vi "choosePlayVSS.vi"(8 "error in (no error)":errorcluster, 11 "Game in":refnum<class "Game.lvclass">) -> (0 "error out":errorcluster, 3 "Game out":refnum<class "Game.lvclass">)   [LabVIEW 2018, in "Game.lvclass"]
uses:
  Game.lvclass
  Referee_class/command_interpreted.ctl
  Game.lvclass/Game.ctl
  Referee_class/Referee.lvclass/Referee.ctl
  HaltPlay_class/HaltPlay.lvclass
  PreparePenaltyAllyPlayVSS_class/PreparePenaltyAllyPlayVSS.lvclass
  Read KeeperTeam.vi
  Read Referee.vi
  Referee_class/Read command_interpreted.vi
  Read AllyRef.vi
  Write AllyRef.vi
  Write KeeperTeam.vi
  Ally_class/Ally.lvclass
  C:/Users/anton/Desktop/RoboIme/vsspssl/SSL_AI/Team_class/Team.lvclass
  Referee_class/Referee.lvclass
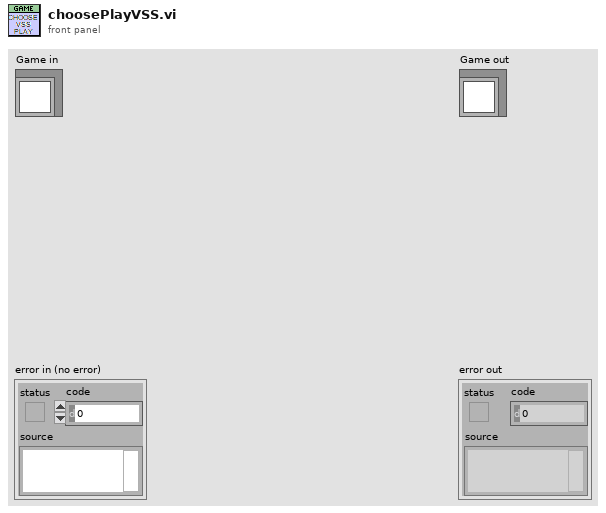
[diagram p1: front panel]
types:
  T1 = typedef "command_interpreted.ctl" = enum16{"Goal Ally", "Goal Enemy", "Ball Placement Enemy", "Ball Placement Ally", "Normal Half Time", "Extra Time  Break", "Extra Half Time", "None", "Post Game", "PKA Normal Start", "Prepare Kickoff Ally", "PKE Normal Start", "Prepare Kickoff Enemy", "Force Start", "Halt", "Timeout", "Prepare Penalty Ally", "Prepare Penalty Enemy", "PPA NormalStart", "PPE Normal Start", "Indirect Free Ally", "Direct Free Enemy", "Direct Free Ally", "Indirect Free Enemy", "Stop"}
  T2 = enum16{"Timeout", "NormalGame", "KickPenaltyAlly", "PenaltyEnemy", "BallChallenge", "PreparePenaltyAlly", "Halt"}
  T3 = enum16{"Timeout", "NormalGame", "KickPenaltyAlly", "PenaltyEnemy", "BallChallenge", "PreparePenaltyAlly", "Halt"}[]
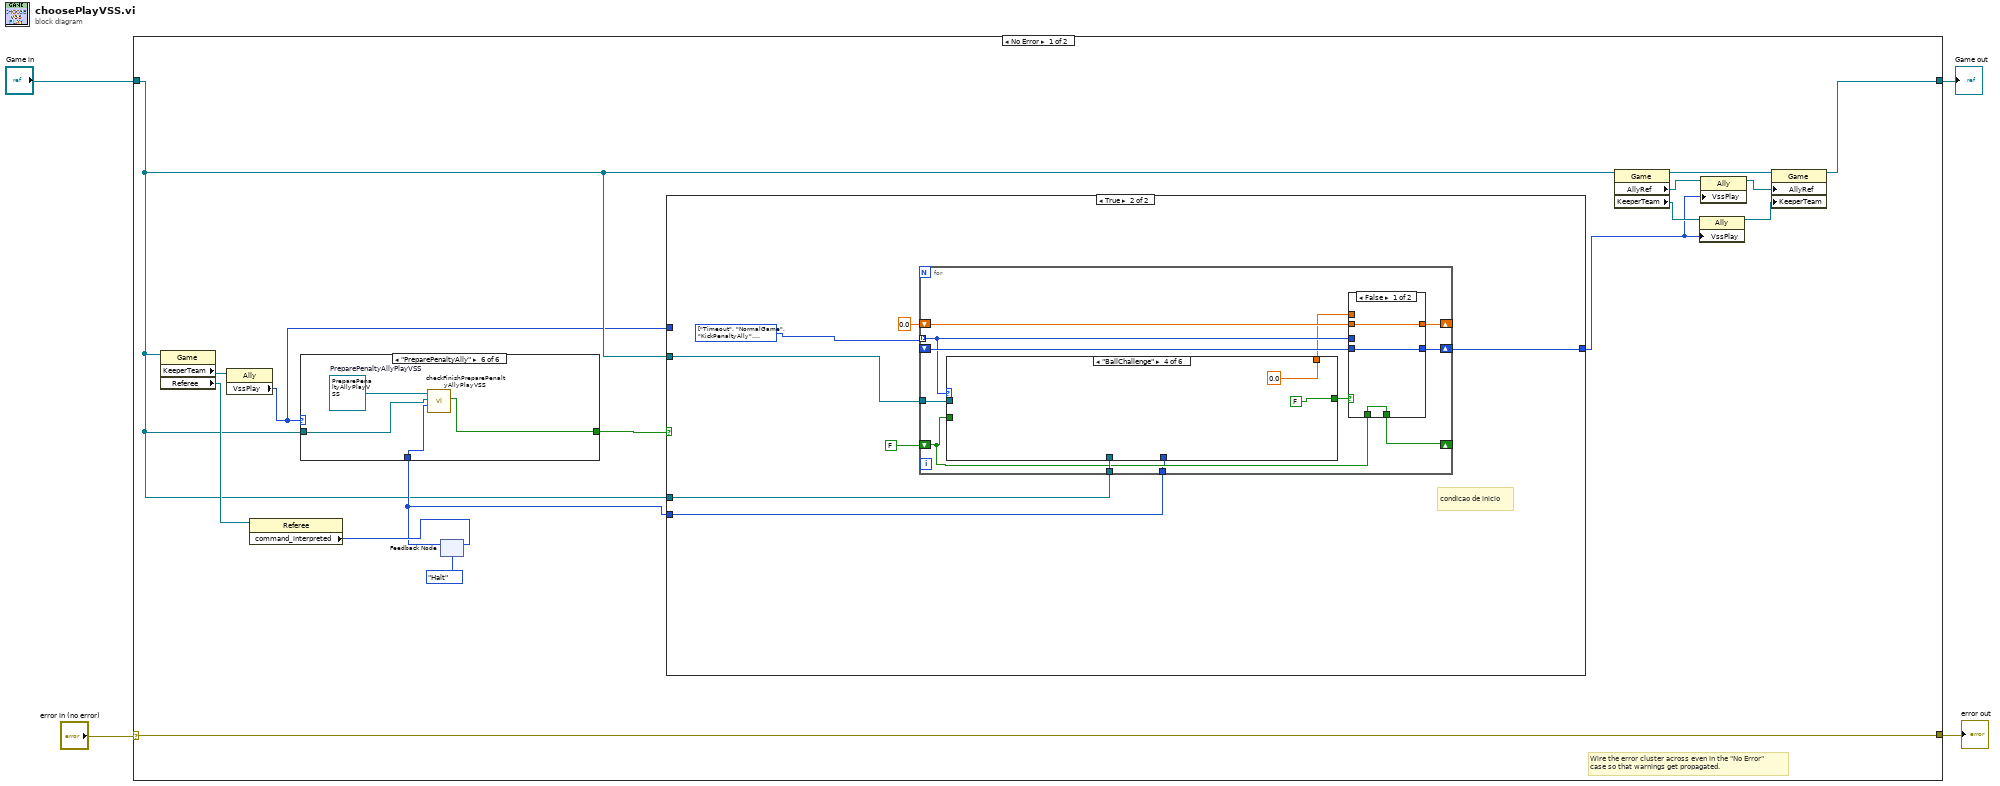
[diagram p0: block diagram]
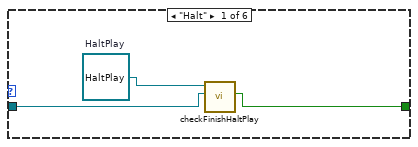
[diagram p2: hidden frame]
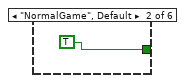
[diagram p3: hidden frame]
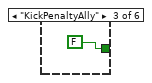
[diagram p4: hidden frame]
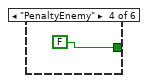
[diagram p5: hidden frame]
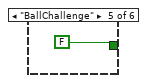
[diagram p6: hidden frame]
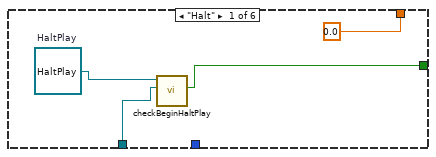
[diagram p8: hidden frame]
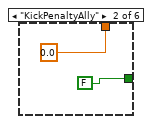
[diagram p9: hidden frame]
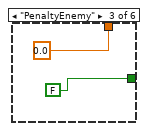
[diagram p10: hidden frame]
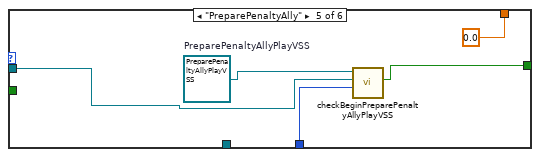
[diagram p11: hidden frame]
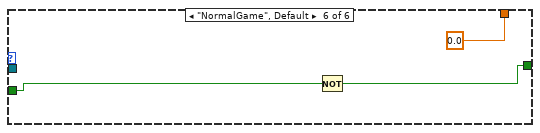
[diagram p12: hidden frame]
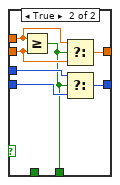
[diagram p13: hidden frame]
diagram:
  n1 = case shown="No Error" "error in (no error)" {
    selector: "error in (no error)" -> [w20 w81]
    tunnel: [w20 w81] -> w3
    tunnel: [w18 w80] -> w1
    tunnel: "Game in" -> [w7 w80]
    frame No Error {
      # "Wire the error cluster across even in the \"No Error\"\ncase so that warnings get propagated."
      n2 = property class="Game"(reference=w7) -> ("KeeperTeam"=w6:refnum<class "Ally.lvclass">, "Referee"=w11:refnum<class "Referee.lvclass">)  [unwired: 1 in, 2 out]
      n3 = property class="Ally"(reference=w6) -> ("VssPlay"=w5:T2)  [unwired: 1 in, 2 out]
      n4 = property class="Referee"(reference=w11) -> ("command_interpreted"=w10:T1)  [unwired: 1 in, 2 out]
      n5 = feedback-in #1(w10) -> ()
      n6 = feedback #1(command_interpreted."Halt" ("command_interpreted")) -> (w8:T1)
      n7 = case shown="\"PreparePenaltyAlly\"" w5 {
        tunnel: [w21 TRUE FALSE FALSE FALSE w28] -> w17
        tunnel: w7 -> [w22 _ _ _ _ w30]
        tunnel: w8 -> [_ _ _ _ _ w29]
        frame "Halt" {
          w23 = refnum<class "HaltPlay.lvclass"> refnum  # HaltPlay
          n8 = call "checkFinishHaltPlay.vi"("Game"=w22, "HaltPlay in"=w23) -> ("Boolean"=w21:bool)  [unwired: 7 in, 2 out]
        }
        frame "NormalGame", Default {
        }
        frame "KickPenaltyAlly" {
        }
        frame "PenaltyEnemy" {
        }
        frame "BallChallenge" {
        }
        frame "PreparePenaltyAlly" {
          w31 = refnum<class "PreparePenaltyAllyPlayVSS.lvclass"> refnum  # PreparePenaltyAllyPlayVSS
          n9 = call "checkFinishPreparePenaltyAllyPlayVSS.vi"("last command_interpreted"=w29, "Game"=w30, "PreparePenaltyAllyPlayVSS in"=w31) -> ("Boolean"=w28:bool)  [unwired: 6 in, 2 out]
        }
      }
      n10 = case shown="True" w17 {
        tunnel: [w32 w38] -> w12
        tunnel: w5 -> [w32 _]
        tunnel: w7 -> [_ w37]
        tunnel: w8 -> [_ w35]
        tunnel: w7 -> [_ w34]
        frame False {
        }
        frame True {
          w33 = T3 [enum."Timeout", enum."NormalGame", enum."KickPenaltyAlly", enum."PenaltyEnemy", enum."BallChallenge", enum."PreparePenaltyAlly", enum."Halt"] items=["Timeout", "NormalGame", "KickPenaltyAlly", "PenaltyEnemy", "BallChallenge", "PreparePenaltyAlly", "Halt"] ("VssPlay")
          # "condicao de inicio"
          n11 = for {
            tunnel: w33 -> [w47] mode=indexing
            shift-right: [w50] -> _
            shift-left: 0.0 -> [w49]
            shift-right: [w48] -> w38
            shift-left: _ -> [w51]
            tunnel: w37 -> [w44]
            shift-right: [w43] -> _
            shift-left: FALSE -> [w42]
            tunnel: w35 -> [w41]
            tunnel: w34 -> [w40]
            n12 = case shown="\"BallChallenge\"" w47 {
              tunnel: [w53 FALSE FALSE FALSE w63 w69] -> w46
              tunnel: [0.0 0.0 0.0 0.0 0.0 0.0] -> w45
              tunnel: w44 -> [w54 _ _ _ _ _]
              tunnel: w42 -> [_ _ _ _ _ w68]
              tunnel: w41 -> [_ _ _ _ w65 _]
              tunnel: w40 -> [_ _ _ _ w64 _]
              frame "Halt" {
                w55 = refnum<class "HaltPlay.lvclass"> refnum  # HaltPlay
                n13 = call "checkBeginHaltPlay.vi"("Game"=w54, "HaltPlay in"=w55) -> ("Boolean"=w53:bool)  [unwired: 7 in, 2 out]
              }
              frame "KickPenaltyAlly" {
              }
              frame "PenaltyEnemy" {
              }
              frame "BallChallenge" {
              }
              frame "PreparePenaltyAlly" {
                w66 = refnum<class "PreparePenaltyAllyPlayVSS.lvclass"> refnum  # PreparePenaltyAllyPlayVSS
                n14 = call "checkBeginPreparePenaltyAllyPlayVSS.vi"("last command_interpreted"=w65, "Game"=w64, "PreparePenaltyAllyPlayVSS in"=w66) -> ("Boolean"=w63:bool)  [unwired: 6 in, 2 out]
              }
              frame "NormalGame", Default {
                n15 = Not(x=w68) -> (.not. x?=w69:bool)
              }
            }
            n16 = case shown="False" w46 {
              tunnel: w51 -> [w71 w76]
              tunnel: [w72 w79] -> w50
              tunnel: w49 -> [w72 w75]
              tunnel: w47 -> [_ w77]
              tunnel: [w71 w78] -> w48
              tunnel: w45 -> [_ w74]
              tunnel: [w70 w73] -> w43
              tunnel: w42 -> [w70 _]
              frame False {
              }
              frame True {
                n17 = Greater Or Equal?(x=w74, y=w75) -> (x >= y?=w73:bool)
                n18 = Select(t=w74, s=w73, f=w75) -> (s? t:f=w79:dbl)
                n19 = Select(t=w77, s=w73, f=w76) -> (s? t:f=w78:T2)
              }
            }
          }
        }
      }
      n20 = property class="Game"(reference=w7) -> (reference out=w19:refnum<class "Game.lvclass">, "AllyRef"=w14:refnum<class "Ally.lvclass">, "KeeperTeam"=w16:refnum<class "Ally.lvclass">)  [unwired: 1 in, 1 out]
      n21 = property class="Ally"(reference=w16, "VssPlay"=w12) -> (reference out=w15:refnum<class "Ally.lvclass">)  [unwired: 1 in, 1 out]
      n22 = property class="Ally"(reference=w14, "VssPlay"=w12) -> (reference out=w13:refnum<class "Ally.lvclass">)  [unwired: 1 in, 1 out]
      n23 = property class="Game"(reference=w19, "AllyRef"=w13, "KeeperTeam"=w15) -> (reference out=w18:refnum<class "Game.lvclass">)  [unwired: 1 in, 1 out]
    }
    frame Error {
    }
  }
  "error out" <- w3
  "Game out" <- w1
